vi "MessageFlag.vi"(10 "Id":u32, 11 "event":bool=TRUE) -> (2 "Array":u8[](array[numeric]))   [LabVIEW 2017]
uses:
  Varint Encoder uint32.vi
panel:
  in  "Array In":u8[](array[numeric])
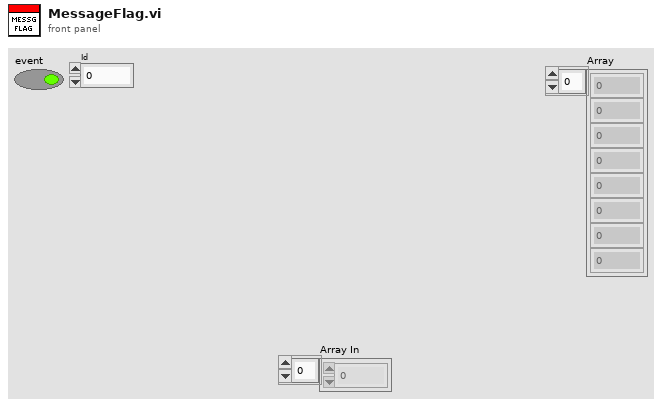
[diagram p1: front panel]
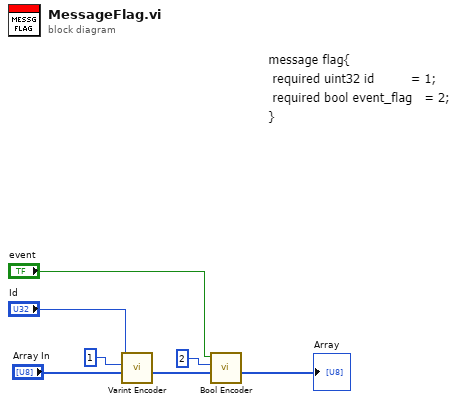
[diagram p0: block diagram]
diagram:
  n1 = call-poly "Varint Encoder.vi"("Array In"="Array In", "Key"=u32 1, "Value"="Id") -> ("Array"=w5:u8[])  [unwired: 8 in]
  n2 = call "Bool Encoder.vi"("Array In"=w5, "Key"=u32 2, "Value"="event") -> ("Array"=→"Array":u8[])  [unwired: 8 in]
